vi "Move and Wait.vi"(4 "error IO":errorcluster, 6 "Absolute position":dbl, 7 "Axis":string) -> (0 "error out":errorcluster)   [LabVIEW 2010, in "PI E710 Stage.lvlib"]
uses:
  PI E710 Stage.lvlib
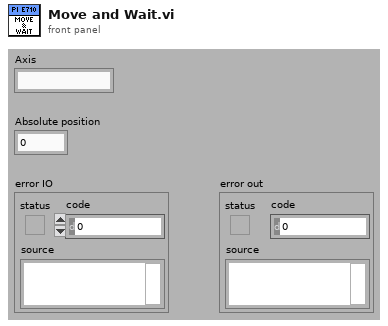
[diagram p1: front panel]
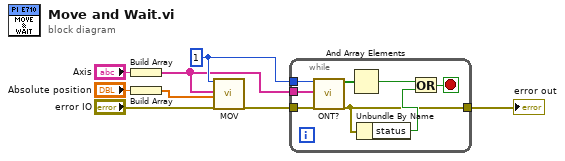
[diagram p0: block diagram]
diagram:
  w3 = 1 ("System no.")
  n1 = Build Array("Axis") -> (w2:string[])
  n2 = Build Array("Absolute position") -> (w5:dbl[])
  n3 = call "MOV.vi"("System no."=w3, "Axes to move"=w2, "Position values"=w5, "error in"="error IO") -> ("error out"=w4:errorcluster)  [unwired: 15 in]
  n4 = while {
    tunnel: w4 -> [w16]
    tunnel: w3 -> [w15]
    tunnel: w2 -> [w14]
    tunnel: [w9] -> w1
    stop <- w12 stop-if-true
    n5 = call "ONT?.vi"("System no."=w15, "Axes to query"=w14, "error in"=w16) -> ("Axis on target?"=w13:bool[], "error out"=w9:errorcluster)  [unwired: 15 in]
    n6 = And Array Elements(Boolean array=w13) -> (logical AND=w11:bool)
    n7 = Unbundle By Name(w9) -> ("status"=w10:bool)
    n8 = Or(x=w11, y=w10) -> (x .or. y?=w12:bool)
  }
  "error out" <- w1
